vi "Find term type by ID.vi"   [LabVIEW 2012, in "Scripting Tools.lvlib" / "XNode Support.lvlib"]
uses:
  XNode Support.lvlib
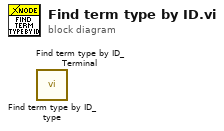
[diagram p0: block diagram]
diagram:
  n1 = call "Find term type by ID_type.vi"() -> ()  [unwired: 7 in, 5 out]
  n2 = call "Find term type by ID_Terminal.vi"() -> ()  [unwired: 7 in, 5 out]
